vi "Actor Core.vi"(8 "error in":errorcluster, 11 "UI in":refnum<class "UI.lvclass">) -> (0 "error out":errorcluster, 3 "Actor out":refnum<class "Actor.lvclass">)   [LabVIEW 2021, in "UI.lvlib" / "UI.lvclass"]
doc: "(<B>Filename</B>: Actor Framework.lvlib:Actor.lvclass:Actor Core.vi)\n\nReceives messages to the actor, reacts to them, and initiates any error handling that may shut the actor down.\n\nDescendant classes may override this VI to append parallel tasks for the actor to complete while it handles messages. Overrides use the Call Parent Class Method node."
uses:
  UI.lvclass
  C:/Program Files (x86)/National Instruments/LabVIEW 2021/vi.lib/ActorFramework/Actor/Actor.lvclass
  <vilib>/ActorFramework/Actor/Actor.lvclass
  UI.lvclass/UI.ctl
  <vilib>/ActorFramework/Actor/Actor.lvclass/Actor.ctl
  <vilib>/ActorFramework/Message Enqueuer/Message Enqueuer.lvclass/Message Enqueuer.ctl
  <vilib>/ActorFramework/Message Enqueuer/Init from Existing Queue.vi
  <vilib>/ActorFramework/Message Enqueuer/Enqueue.vi
  UI Messages/Get Sine Msg/Get Sine Msg.lvclass
  C:/Program Files (x86)/National Instruments/LabVIEW 2021/vi.lib/ActorFramework/Message/Message.lvclass
  <vilib>/ActorFramework/Stop Msg/Stop Msg.lvclass
  <vilib>/ActorFramework/Message Priority Queue/Priority Enqueue.vi
  <vilib>/ActorFramework/Message Enqueuer/Message Enqueuer.lvclass
panel:
  in  "Stop":bool
  out "Waveform Chart":dbl(graph)
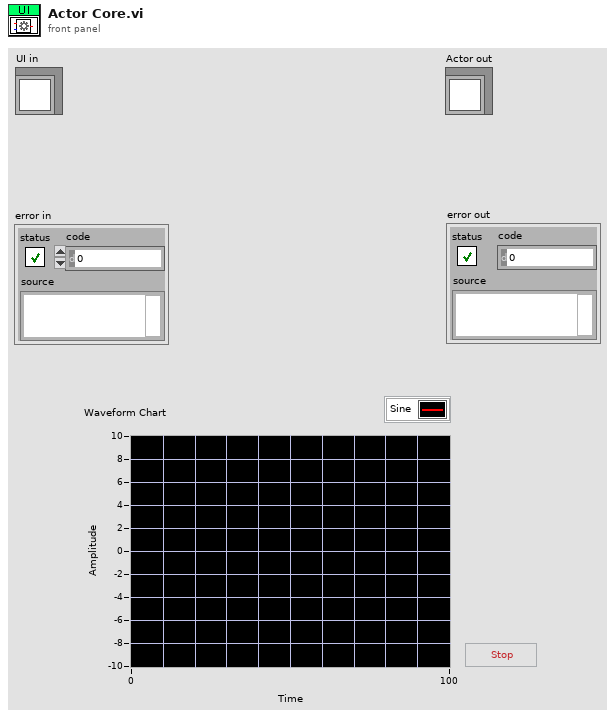
[diagram p1: front panel]
types:
  T1 = enum32{"Invalid", "Standard", "Closed", "Hidden", "Minimized", "Maximized"}
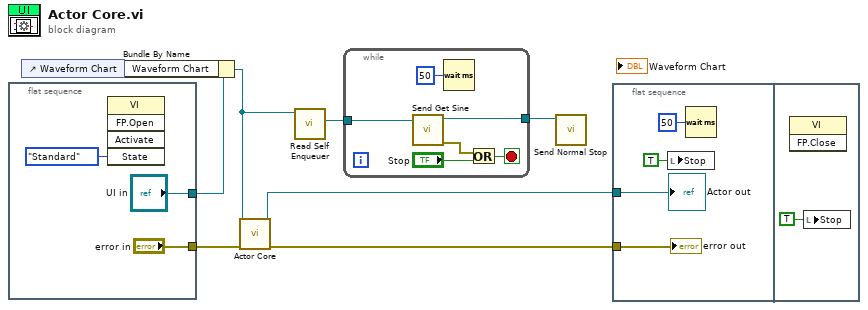
[diagram p0: block diagram]
diagram:
  n1 = flat-sequence {
    tunnel: ["UI in"] -> w4
    tunnel: ["error in"] -> w6
    frame #0 {
      n2 = invoke class="VI" method="FP.Open"("State"=T1."Standard") -> ()  [unwired: 4 in, 5 out]
    }
  }
  n3 = control-ref of="Waveform Chart"() -> (w5:refnum<vi>)
  n4 = Bundle By Name(cluster=w4, "Waveform Chart"=w5) -> (w2:refnum<class "UI.lvclass">)
  n5 = call-parent "Actor Core.vi"("error in"=w6, "Actor in"=w2) -> ("error out"=w8:errorcluster, "Actor out"=w7:refnum<class "Actor.lvclass">)  [unwired: 8 in]
  n6 = call <vilib>:"Read Self Enqueuer.vi"("Actor"=w2) -> ("Self Enqueuer"=w3:refnum<class "Message Enqueuer.lvclass">)  [unwired: 10 in]
  n7 = while {
    tunnel: w3 -> [w16]
    tunnel: [w12] -> w1
    stop <- w13 stop-if-true
    n8 = call "Send Get Sine.vi"("Message Enqueuer"=w16) -> ("error out"=w15:errorcluster, "Message Enqueuer out"=w12:refnum<class "Message Enqueuer.lvclass">)  [unwired: 9 in]
    n9 = Wait (ms)(milliseconds to wait=u32 50) -> ()  [unwired: 1 out]
    n10 = Or(x=w15, y="Stop") -> (x .or. y?=w13:bool)
  }
  n11 = call <vilib>:"Send Normal Stop.vi"("Message Enqueuer"=w1) -> ()  [unwired: 10 in, 1 out]
  n12 = flat-sequence {
    tunnel: w8 -> [w21]
    tunnel: w7 -> [w20]
    frame #0 {
      n13 = local write "Stop"(TRUE ("Stop")) -> ()
      n14 = Wait (ms)(milliseconds to wait=u32 50) -> ()  [unwired: 1 out]
      "error out" <- w21
      "Actor out" <- w20
    }
    frame #1 {
      n15 = invoke class="VI" method="FP.Close"() -> ()  [unwired: 3 in, 3 out]
      n16 = local write "Stop"(TRUE ("Stop")) -> ()
    }
  }
